vi "Send_RC_Switch_directDACmx_fail.vi"() -> ()   [LabVIEW 2016]
uses:
  <vilib>/DAQmx/write.llb/DAQmx Write (Digital Bool 1Line 1Point).vi
  <vilib>/DAQmx/create/channels.llb/DAQmx Create Channel (DO-Digital Output).vi
  <vilib>/DAQmx/configure/timing.llb/DAQmx Timing (Sample Clock).vi
  <vilib>/DAQmx/miscellaneous.llb/DAQmx Fill In Error Info.vi
panel:
  in  "auto start":bool=TRUE
  out "Numeric 2":i32
  in  "Numeric":i32
  in  "send":bool
  in  "pulse-length (us)":dbl=1000.0 format="%0.2f"
  in  "stop":bool
  in  "error in":errorcluster
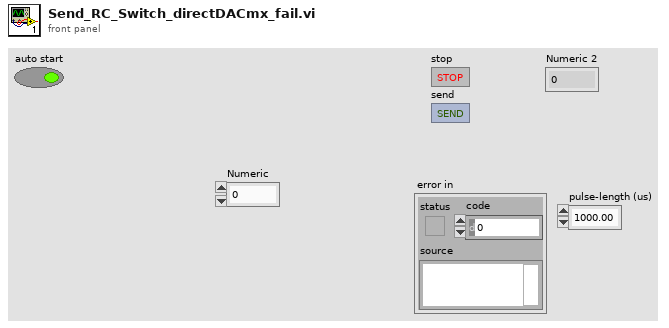
[diagram p1: front panel]
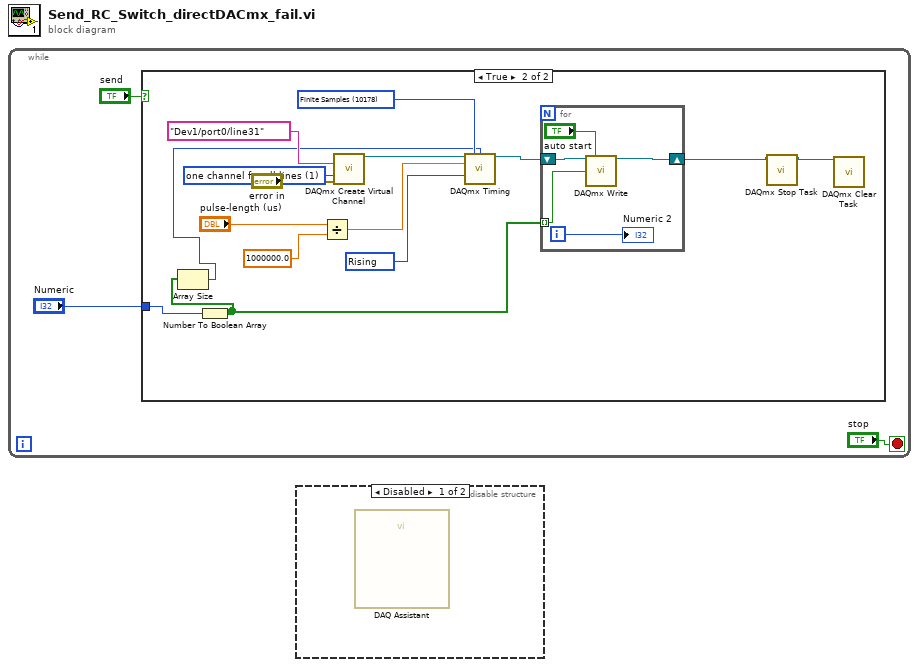
[diagram p0: block diagram]
diagram:
  n1 = while {
    stop <- "stop" stop-if-true
    n2 = case shown="True" "send" {
      tunnel: "Numeric" -> [_ w7]
      frame False {
      }
      frame True {
        w9 = 1 items=["one channel for each line", "one channel for all lines"] ("line grouping")
        w14 = 10178 items=["Finite Samples"=10178, "Continuous Samples"=10123, "Hardware Timed Single Point"=12522] ("sample mode")
        w13 = 10280 items=["Rising"=10280, "Falling"=10171] ("active edge")
        n3 = Number To Boolean Array(number=w7) -> (Boolean array=w4:bool[])
        n4 = Array Size(array=w4) -> (size(s)=w8:i32)
        n5 = Divide(x="pulse-length (us)", y=1000000.0) -> (x/y=w12:dbl)
        n6 = call-poly <vilib>:"DAQmx Create Virtual Channel.vi"("lines"=tag "Dev1/port0/line31", "line grouping"=w9, "error in"="error in") -> ("task out"=w16:refnum<k21>)  [unwired: 11 in, 1 out]
        n7 = call-poly <vilib>:"DAQmx Timing.vi"("task/channels in"=w16, "sample mode"=w14, "samples per channel"=w8, "rate"=w12, "active edge"=w13) -> ("task out"=w15:refnum<k21>)  [unwired: 9 in, 1 out]
        n8 = for {
          shift-right: [w22] -> w6
          shift-left: w15 -> [w23]
          tunnel: w4 -> [w21] mode=indexing
          i -> [w20]
          n9 = call-poly <vilib>:"DAQmx Write.vi"("task/channels in"=w23, "auto start"="auto start", "data"=w21) -> ("task out"=w22:refnum<k21>)  [unwired: 10 in, 2 out]
          "Numeric 2" <- w20
        }
        n10 = call <vilib>:"DAQmx Stop Task.vi"("task/channels in"=w6) -> ("task out"=w5:refnum<k21>)  [unwired: 13 in, 1 out]
        n11 = call <vilib>:"DAQmx Clear Task.vi"("task in"=w5) -> ()  [unwired: 14 in, 1 out]
      }
    }
  }
  n12 = disable-structure shown="Disabled" {
    frame Disabled {
      n13 = call "DAQ Assistant"() -> ()  [unwired: 18 in, 2 out]
    }
    frame Enabled {
    }
  }
